vi "Run Tests.vi"(8 "error in (no error)":errorcluster) -> (0 "error out":errorcluster)   [LabVIEW 2015]
uses:
  <vilib>/addons/_JKI Toolkits/Caraya/classes/Test Suite/Test Suite.lvclass
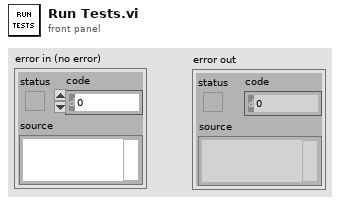
[diagram p1: front panel]
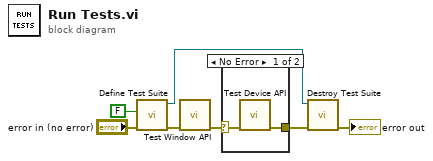
[diagram p0: block diagram]
diagram:
  n1 = call <vilib>:"Define Test Suite.vi"("error in (no error)"="error in (no error)", "Interactive"=FALSE) -> ("error out"=w3:errorcluster, "Test Suite"=w6:refnum<class "Test Suite.lvclass">)  [unwired: 8 in]
  n2 = call "Test Window API.vi"("error in (no error)"=w3) -> ("error out"=w4:errorcluster)  [unwired: 10 in]
  n3 = case shown="No Error" w4 {
    selector: w4 -> [w8 w10]
    tunnel: [w9 w10] -> w2
    frame No Error {
      n4 = call "Test Device API.vi"("error in (no error)"=w8) -> ("error out"=w9:errorcluster)  [unwired: 10 in]
    }
    frame Error {
    }
  }
  n5 = call-dynamic "Destroy Test Suite.vi"("error in (no error)"=w2, "Test Suite in"=w6) -> ("error out"=→"error out":errorcluster)  [unwired: 9 in]
